vi "Engine.vi"(0 "object in":refnum<class "MTEC_Async.lvclass">, 2 "Sample Rate (Hz)":dbl=10.0 format="%#_13g", 5 "error in (no error)":errorcluster) -> (14 "object out":refnum<class "MTEC_Async.lvclass">, 19 "error out":errorcluster)   [LabVIEW 2019, in "MTEC_Async.lvclass"]
uses:
  MTEC_Async.lvclass
  MTEC_Async.lvclass/MTEC_Async.ctl
  TEC LabVIEW Control Software v0.14/Source/LV Source/[meerstetter engineering TE Cooling]/TypeDefs/meTEC_ID 2000_Input Selection.ctl
  TEC LabVIEW Control Software v0.14/Source/LV Source/[meerstetter engineering TE Cooling]/TypeDefs/meTEC_ID 50011_Object Target Temperature Source Selection.ctl
  TEC LabVIEW Control Software v0.14/Source/LV Source/[meerstetter engineering TE Cooling]/TypeDefs/meTEC_ID 50000_Live Enable.ctl
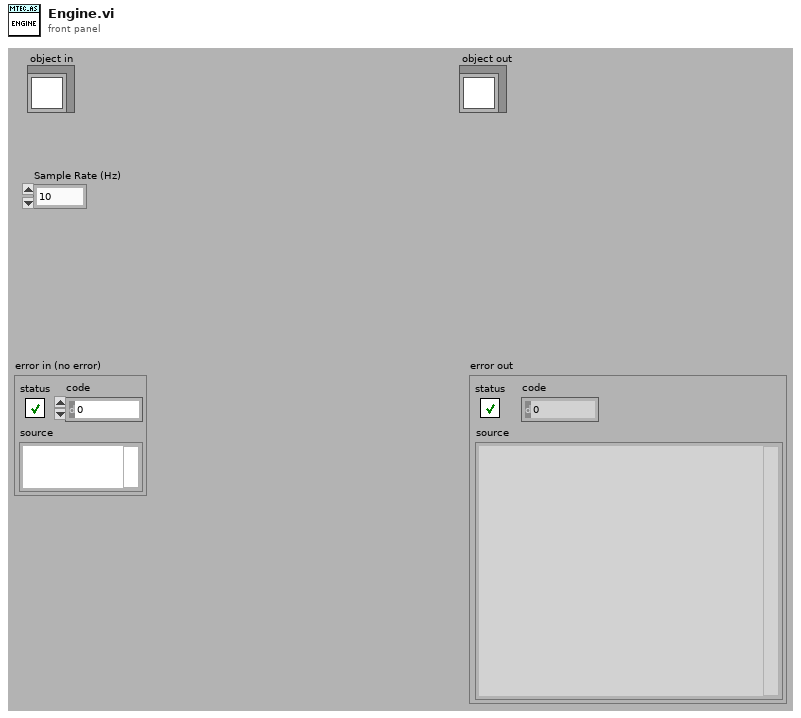
[diagram p1: front panel]
types:
  T1 = typedef "meTEC_ID 2000_Input Selection.ctl" = i32
  T2 = typedef "meTEC_ID 50011_Object Target Temperature Source Selection.ctl" = i32
  T3 = typedef "meTEC_ID 50000_Live Enable.ctl" = i32
  T4 = cluster{"meTEC_CH1_Input Selection (ID 2000)":T1, "meTEC_CH2_Input Selection (ID 2000)":T1, "meTEC_CH1_Object Target Temp. Source Selection (ID 50011)":T2, "meTEC_CH2_Object Target Temp. Source Selection (ID 50011)":T2, "meTEC_CH1_Live Enable (ID 50000)":T3, "meTEC_CH2_Live Enable (ID 50000)":T3, "meTEC_CH1_Object Target Temperature (ID 3000 / 50012) [°C]":dbl, "meTEC_CH2_Object Target Temperature (ID 3000 / 50012) [°C]":dbl, "meTEC_CH1_Live Set Current (ID 50001) [A]":dbl, "meTEC_CH2_Live Set Current (ID 50001) [A]":dbl, "meTEC_CH1_Live Set Voltage (ID 50002) [V]":dbl, "meTEC_CH2_Live Set Voltage (ID 50002) [V]":dbl}
  T5 = cluster{"Message":string, "Message Data":variant}
  T6 = typedef "FGV_TE Controller.ctl" = cluster{"SVs":cluster{"Unused":dbl}, "PVs":cluster{"FW & HW Versions":cluster{"Device Type [I32]":i32, "Device Type [String]":string, "Firmware Version [I32]":i32, "Firmware Version [String]":string, "Hardware Version [I32]":i32, "Hardware Version [String]":string, "Serial No.":i32}, "TEC Configuration":T7, "Object Target Temperature Source_CH1":u8, "Object Target Temperature Source_CH2":u8}, "Front Panel References":T8}
  T7 = typedef "meTEC_Configuration.ctl" = cluster{"VISA resource name":refnum<visa-resource-name>, "Device Address":u16}
  T8 = typedef "FGV_Front Panel References.ctl" = cluster{"Main Loop Queue":refnum<queue>, "meTEC_Device Type":refnum<vi>, "meTEC_Serial No.":refnum<vi>, "meTEC_Hardware Version":refnum<vi>, "meTEC_Firmware Version":refnum<vi>, "meTEC_CH1_Object Target Temperature (ID 3000 / 50012) [°C]":refnum<vi>, "meTEC_CH1_Live Set Current (ID 50001) [A]":refnum<vi>, "meTEC_CH1_Live Set Voltage (ID 50002) [V]":refnum<vi>, "meTEC_CH1_Live Enable (ID 50000)":refnum<vi>, "meTEC_CH1_Input Selection (ID 2000)":refnum<vi>, "meTEC_CH1_Object Target Temp. Source Sel. (ID 50011)":refnum<vi>, "meTEC_CH2_Object Target Temperature (ID 3000 / 50012) [°C]":refnum<vi>, "meTEC_CH2_Live Set Current (ID 50001) [A]":refnum<vi>, "meTEC_CH2_Live Set Voltage (ID 50002) [V]":refnum<vi>, "meTEC_CH2_Live Enable (ID 50000)":refnum<vi>, "meTEC_CH2_Input Selection (ID 2000)":refnum<vi>, "meTEC_CH2_Object Target Temp. Source Sel. (ID 50011)":refnum<vi>, "meTEC_CH2_Object Temperature [°C]":refnum<vi>, "meTEC_CH2_Sink Temperature [°C]":refnum<vi>, "meTEC_CH2_Act. Output Current [A]":refnum<vi>, "meTEC_CH2_Act. Output Voltage [V]":refnum<vi>, "meTEC_CH2_Temperature Stability":refnum<vi>, "Monitor Chart_CH2":refnum<vi>, "meTEC_Initialize Device":refnum<vi>}
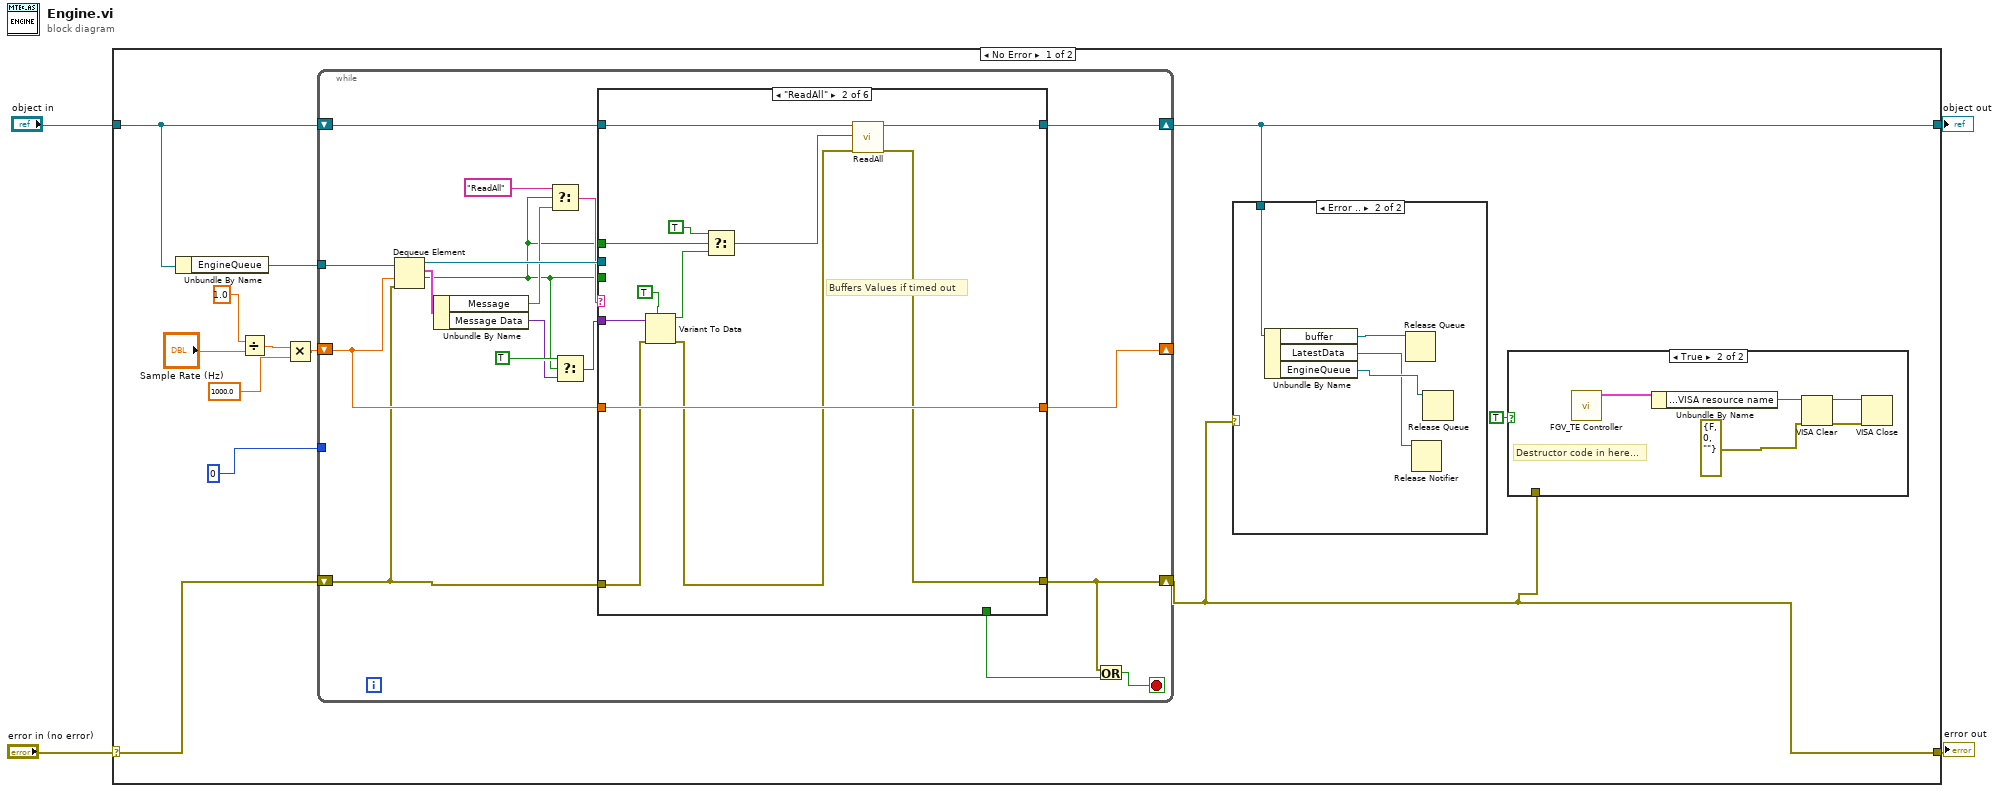
[diagram p0: block diagram]
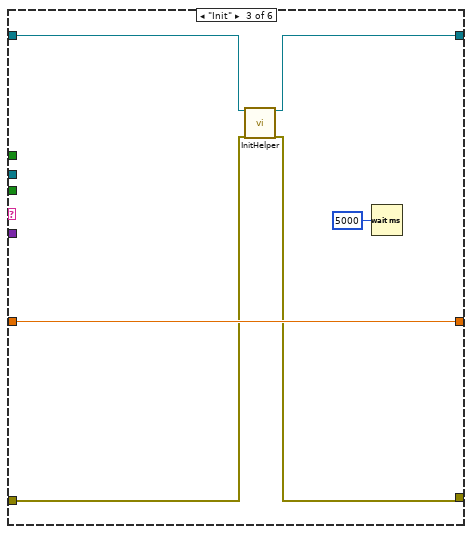
[diagram p5: hidden frame]
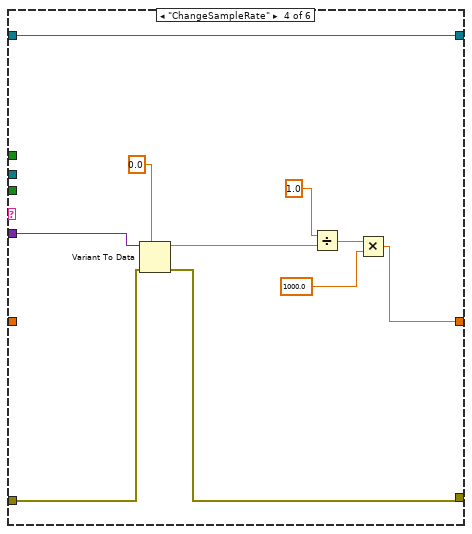
[diagram p6: hidden frame]
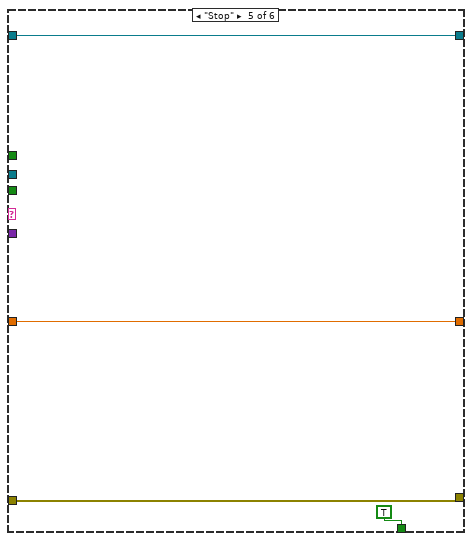
[diagram p7: hidden frame]
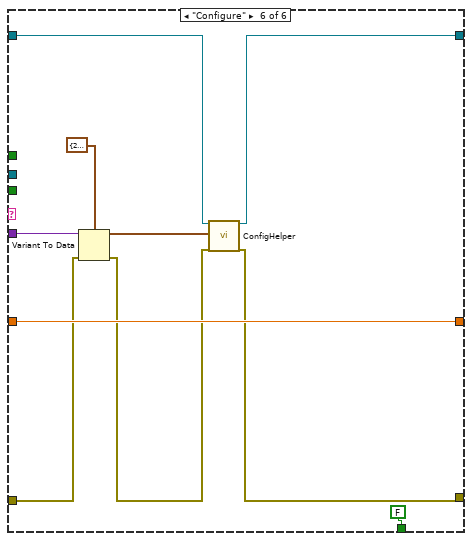
[diagram p8: hidden frame]
diagram:
  n1 = case shown="No Error" "error in (no error)" {
    selector: "error in (no error)" -> [w9 w90]
    tunnel: [w6 w90] -> w3
    tunnel: [w7 w89] -> w1
    tunnel: "object in" -> [w16 w89]
    frame No Error {
      n2 = Unbundle By Name(w16) -> ("EngineQueue"=w8:refnum<queue>)
      n3 = Divide(x=1.0, y="Sample Rate (Hz)") -> (x/y=w12:dbl)
      n4 = Multiply(x=w12, y=1000.0) -> (x*y=w10:dbl)
      n5 = while {
        shift-right: [w37] -> w7
        shift-left: w16 -> [w38]
        tunnel: w8 -> [w43]
        shift-right: [w40] -> w6
        shift-left: w9 -> [w26]
        tunnel: u32 0 ("millisecond multiple") -> [_]
        shift-right: [w36] -> _
        shift-left: w10 -> [w34]
        stop <- w41 stop-if-true
        n6 = Dequeue Element(queue=w43, timeout in ms (-1)=w34, error in (no error)=w26) -> (queue out=w35:refnum<queue>, element=w42:T5, timed out?=w29:bool)  [unwired: 1 out]
        n7 = Unbundle By Name(w42) -> ("Message"=w31:string, "Message Data"=w28:variant)
        n8 = Select(t="ReadAll", s=w29, f=w31) -> (s? t:f=w33:string)
        n9 = Select(t=TRUE, s=w29, f=w28) -> (s? t:f=w27:variant)
        n10 = case shown="\"ReadAll\"" w33 {
          tunnel: w35 -> [_ _ _ _ _ _]
          tunnel: w26 -> [w46 w52 w60 w71 w78 w81]
          tunnel: [w46 w55 w61 w72 w78 w79] -> w40
          tunnel: [_ _ _ _ TRUE FALSE] -> w39
          tunnel: [w45 w58 w63 w74 w76 w86] -> w37
          tunnel: w38 -> [w45 w57 w62 w74 w76 w85]
          tunnel: w34 -> [w44 w56 w64 _ w75 w87]
          tunnel: [w44 w56 w64 w66 w75 w87] -> w36
          tunnel: w27 -> [_ w54 _ w65 _ w84]
          tunnel: w29 -> [_ _ _ _ _ _]
          tunnel: w29 -> [_ w50 _ _ _ _]
          frame "False", Default {
          }
          frame "ReadAll" {
            # "Buffers Values if timed out"
            n11 = Variant To Data(error in=w52, type=TRUE, Variant=w54) -> (data=w47:bool, error out=w53:errorcluster)
            n12 = Select(t=TRUE, s=w50, f=w47) -> (s? t:f=w48:bool)
            n13 = call-dynamic "ReadAll.vi"("object in"=w57, "Buffer Values?"=w48, "error in (no error)"=w53) -> ("object out"=w58:refnum<class "MTEC_Async.lvclass">, "error out"=w55:errorcluster)  [unwired: 15 in]
          }
          frame "Init" {
            n14 = call-dynamic "InitHelper.vi"("object in"=w62, "error in (no error)"=w60) -> ("object out"=w63:refnum<class "MTEC_Async.lvclass">, "error out"=w61:errorcluster)  [unwired: 16 in]
            n15 = Wait (ms)(milliseconds to wait=u32 5000) -> ()  [unwired: 1 out]
          }
          frame "ChangeSampleRate" {
            n16 = Variant To Data(error in=w71, type=0.0, Variant=w65) -> (data=w67:dbl, error out=w72:errorcluster)
            n17 = Divide(x=1.0, y=w67) -> (x/y=w69:dbl)
            n18 = Multiply(x=w69, y=1000.0) -> (x*y=w66:dbl)
          }
          frame "Stop" {
          }
          frame "Configure" {
            n19 = Variant To Data(error in=w81, type=T4 {"meTEC_CH1_Input Selection (ID 2000)"=2, "meTEC_CH2_Input Selection (ID 2000)"=2, "meTEC_CH1_Object Target Temp. Source Selection (ID 50011)"=0, "meTEC_CH2_Object Target Temp. Source Selection (ID 50011)"=0, "meTEC_CH1_Live Enable (ID 50000)"=0, "meTEC_CH2_Live Enable (ID 50000)"=0, "meTEC_CH1_Object Target Temperature (ID 3000 / 50012) [°C]"=23.0, "meTEC_CH2_Object Target Temperature (ID 3000 / 50012) [°C]"=23.0, "meTEC_CH1_Live Set Current (ID 50001) [A]"=0.0, "meTEC_CH2_Live Set Current (ID 50001) [A]"=0.0, "meTEC_CH1_Live Set Voltage (ID 50002) [V]"=0.0, "meTEC_CH2_Live Set Voltage (ID 50002) [V]"=0.0} ("Config Data"), Variant=w84) -> (data=w82:T4, error out=w80:errorcluster)
            n20 = call-dynamic "ConfigHelper.vi"("object in"=w85, "Config Data"=w82, "error in (no error)"=w80) -> ("object out"=w86:refnum<class "MTEC_Async.lvclass">, "error out"=w79:errorcluster)  [unwired: 15 in]
          }
        }
        n21 = Or(x=w40, y=w39) -> (x .or. y?=w41:bool)
      }
      n22 = case shown="Error .." w6 {
        tunnel: w7 -> [_ w25]
        frame No Error {
        }
        frame Error {
          n23 = Unbundle By Name(w25) -> ("buffer"=w24:refnum<queue>, "LatestData"=w22:refnum<notifier>, "EngineQueue"=w23:refnum<queue>)
          n24 = Release Queue(queue=w24) -> ()  [unwired: 2 in, 3 out]
          n25 = Release Notifier(notifier=w22) -> ()  [unwired: 2 in, 3 out]
          n26 = Release Queue(queue=w23) -> ()  [unwired: 2 in, 3 out]
        }
      }
      n27 = case shown="True" TRUE {
        tunnel: w6 -> [_ _]
        frame False {
        }
        frame True {
          # "Destructor code in here..."
          n28 = call "FGV_TE Controller.vi"() -> ("FGV_TEC_OUT"=w21:T6)  [unwired: 10 in, 1 out]
          n29 = Unbundle By Name(w21) -> ("PVs.TEC Configuration.VISA resource name"=w20:refnum<visa-resource-name>)
          n30 = VISA Clear(VISA resource name=w20, error in (no error)=errorcluster {"status"=FALSE, "code"=0, "source"=""}) -> (VISA resource name out=w19:refnum<visa-resource-name>, error out=w18:errorcluster)
          n31 = VISA Close(VISA resource name=w19, error in (no error)=w18) -> ()  [unwired: 1 out]
        }
      }
    }
    frame Error {
    }
  }
  "error out" <- w3
  "object out" <- w1
